vi "Get Controller Information (Test).vi"() -> (3 "Unit Test Framework Results":T1)   [LabVIEW 2015, in "SMI Tests.lvlib"]
uses:
  SMI Tests.lvlib
  <vilib>/utf/common/utf_test_result_troll.ctl
  <vilib>/utf/common/utf_test_result.ctl
  <vilib>/utf/common/utf_test_result_failure.ctl
  <vilib>/utf/common/utf_test_comparison_operators.ctl
  <vilib>/utf/common/utf_vi_tag.ctl
  classes/SysCfg Device/SysCfg Device.lvclass
  classes/Controller/Controller.lvclass
  <vilib>/utf/NI_UnitTestFramework.lvlib
panel:
  out "error out":errorcluster
  in  "error in":errorcluster
  in  "Device Model":enum16{"cRIO-9068"}(ring)
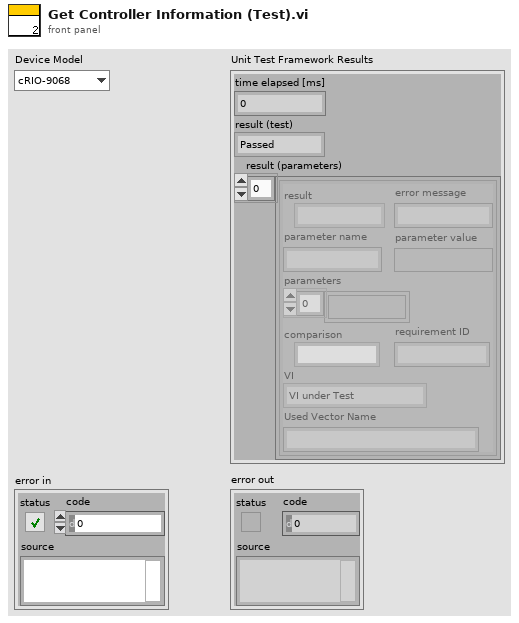
[diagram p1: front panel]
types:
  T1 = typedef "NI_UnitTestFramework.lvlib/utf_test_result_troll.ctl" = cluster{"time elapsed [ms]":u32, "result (test)":T2, "result (parameters)":T3[]}
  T2 = typedef "NI_UnitTestFramework.lvlib/utf_test_result.ctl" = enum16{"Passed", "Failed", "Error", "Skipped", "Not Processed"}
  T3 = typedef "NI_UnitTestFramework.lvlib/utf_test_result_failure.ctl" = cluster{"result":T2, "error message":string, "parameter name":string, "parameter value":variant, "parameters":variant[], "comparison":T4, "requirement ID":string, "VI":T5, "Used Vector Name":string}
  T4 = typedef "NI_UnitTestFramework.lvlib/utf_test_comparison_operators.ctl" = enum16{"=", "!=", ">", ">=", "<", "<=", "range", "symmetric tolerance", "asymmetric tolerance", "string contains", "string not contain", "array size", "string length", "array range", "by element", "array range (limit array)", "user-defined", "array contains", "array not contain", "vector length", "= (elm)", "!= (elm)", "= (case insensitive)", "!= (case insensitive)"}
  T5 = typedef "NI_UnitTestFramework.lvlib/utf_vi_tag.ctl" = enum16{"Setup VI", "VI under Test", "Teardown VI"}
  T6 = typedef "SMI.lvlib/Controller.lvclass/ControllerInformation.ctl" = cluster{"SysCfg Session":refnum<data-value>, "System Hardware Reference":refnum<data-value>, "Vendor Name":string, "Product Name":string, "Product ID":u16, "Serial Number":string, "Device Information":T7, "Primary Network Adapter":T8, "Secondary Network Adapters":T8[]}
  T7 = typedef "SMI.lvlib/Controller.lvclass/DeviceInformation.ctl" = cluster{"Resource":string, "Device Class":string, "System Start Time":timestamp, "Current Time":timestamp, "Time Zone":string, "Firmware Revision":string, "Image Title":string, "Image Version":string, "System Status":string}
  T8 = typedef "SMI.lvlib/Controller.lvclass/NetworkAdapterSettings.ctl" = cluster{"IP Address":string, "MAC Address":string, "IP Address Request Mode":u32, "SubnetMask":string, "Gateway":string, "DNS Server":string, "Adapter Mode":u32, "Adapter Type":u32}
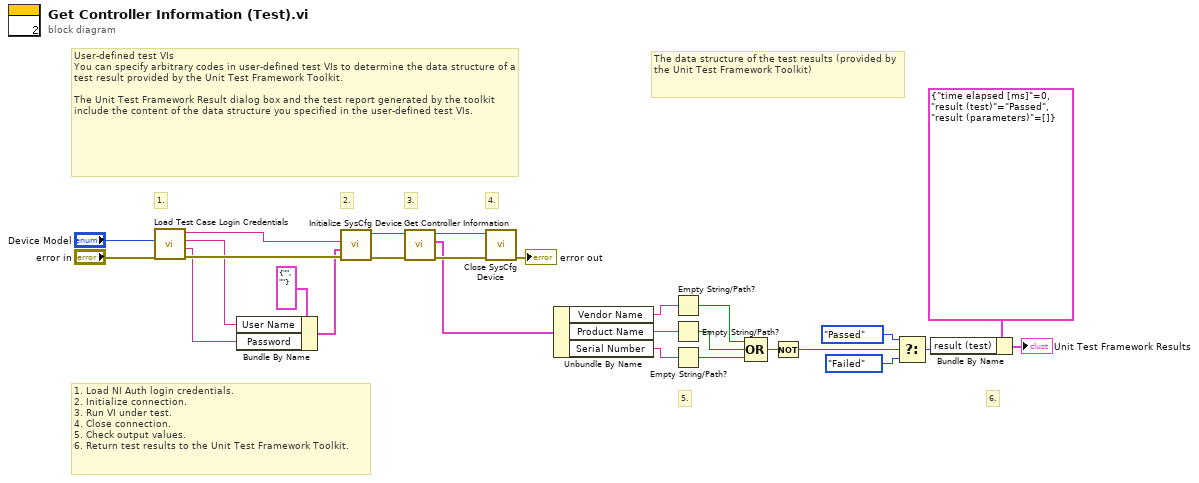
[diagram p0: block diagram]
diagram:
  # "6."
  # "4."
  # "1. Load NI Auth login credentials.\n2. Initialize connection.\n3. Run VI under test.\n4. Close connection.\n5. Check output values.\n6. Return test results to the Unit Test Framework Toolkit."
  # "2."
  # "1."
  # "3."
  # "User-defined test VIs\nYou can specify arbitrary codes in user-defined test VIs to determine the data structure of a test result provided by the Unit Test Framework Toolkit.\n\nThe Unit Test Framework Result dialog box and the test report generated by the toolkit include the content of the data structure you specified in the user-defined test VIs."
  # "The data structure of the test results (provided by the Unit Test Framework Toolkit)"
  # "5."
  n1 = call "Load Test Case Login Credentials.vi"("error in"="error in", "Device Model"="Device Model") -> ("error out"=w27:errorcluster, "Password"=w22:string, "Username"=w23:string, "IP Address"=w21:string)  [unwired: 6 in]
  n2 = Bundle By Name(cluster=cluster{"User Name":string, "Password":string} {"User Name"="", "Password"=""} ("NI Auth (Unconfigured)"), "User Name"=w23, "Password"=w22) -> (w20:cluster{"User Name":string, "Password":string})
  n3 = call "Initialize SysCfg Device.vi"("error in"=w27, "NI Auth (Unconfigured)"=w20, "Target Address"=w21) -> ("error out"=w26:errorcluster, "Controller out"=w19:refnum<class "Controller.lvclass">)  [unwired: 7 in]
  n4 = call "Get Controller Information.vi"("error in"=w26, "Controller in"=w19) -> ("error out"=w25:errorcluster, "Device Information"=w10:T6, "Controller out"=w18:refnum<class "Controller.lvclass">)  [unwired: 7 in]
  n5 = call "Close SysCfg Device.vi"("error in"=w25, "Controller in"=w18) -> ("error out"=→"error out":errorcluster)  [unwired: 9 in]
  n6 = Unbundle By Name(w10) -> ("Vendor Name"=w7:string, "Product Name"=w6:string, "Serial Number"=w9:string)
  n7 = Empty String/Path?(string/path=w7) -> (empty?=w5:bool)
  n8 = Empty String/Path?(string/path=w6) -> (empty?=w4:bool)
  n9 = Empty String/Path?(string/path=w9) -> (empty?=w3:bool)
  n10 = Compound Arithmetic op=OR(w5, w4, w3) -> (w2:bool)
  n11 = Not(x=w2) -> (.not. x?=w1:bool)
  n12 = Select(t=utf_test_result."Passed" ("Result (Test)"), s=w1, f=utf_test_result."Failed" ("Result (Test)")) -> (s? t:f=w14:T2)
  n13 = Bundle By Name(cluster=T1 {"time elapsed [ms]"=0, "result (test)"=enum."Passed", "result (parameters)"=[]} ("Constant"), "result (test)"=w14) -> (→"Unit Test Framework Results":T1)
